vi "Read Coordinates.CAD Cluster.vi"(8 "error in (no error)":errorcluster, 11 "Sensor Dispense in":refnum<class "Sensor Dispense.lvclass">) -> (0 "error out":errorcluster, 2 "Coordinates.CAD Cluster":T1(array[cluster]), 3 "Sensor Dispense out":refnum<class "Sensor Dispense.lvclass">)   [LabVIEW 2018, in "Sensor Dispense.lvclass"]
uses:
  Projects/Sensor Dispense.lvclass
  Projects/Sensor Dispense.lvclass/Sensor Dispense.ctl
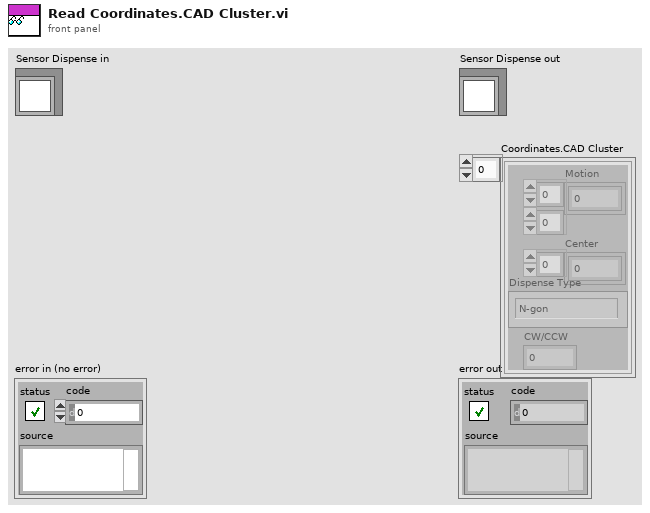
[diagram p1: front panel]
types:
  T1 = cluster{"Motion":dbl[][], "Center":dbl[], "CW/CCW":dbl, "Dispense Type":enum16{"N-gon", "Square", "Arc", "Dot", "Line", "Circle"}}[]
  T2 = cluster{"Endpoints":dbl[][], "Center":dbl[], "CW/CCW":dbl, "Dispense Type":enum16{"N-gon", "Square", "Arc", "Dot", "Line", "Circle"}}[]
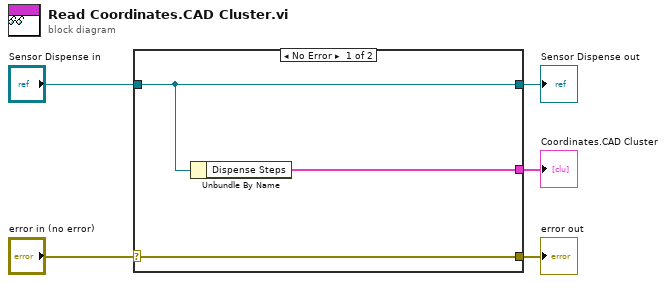
[diagram p0: block diagram]
diagram:
  n1 = case shown="No Error" "error in (no error)" {
    selector: "error in (no error)" -> [w8 w9]
    tunnel: [w8 w9] -> w4
    tunnel: [w7 w10] -> w2
    tunnel: "Sensor Dispense in" -> [w7 w10]
    tunnel: [w6 _] -> w1
    frame No Error {
      n2 = Unbundle By Name(w7) -> ("Dispense Steps"=w6:T2)
    }
    frame Error {
    }
  }
  "error out" <- w4
  "Sensor Dispense out" <- w2
  "Coordinates.CAD Cluster" <- w1
